vi "create.vi"(11 "tasks":refnum<class "task.lvclass">[](array[class])) -> (3 "sequence task out":refnum<class "sequence task.lvclass">)   [LabVIEW 2014, in "sequence task.lvclass"]
uses:
  sequence task.lvclass
  task/task.lvclass
  sequence task.lvclass/sequence task.ctl
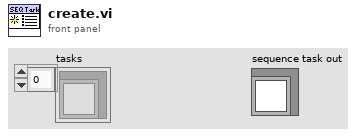
[diagram p1: front panel]
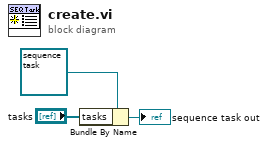
[diagram p0: block diagram]
diagram:
  n1 = Bundle By Name(cluster=refnum<class "sequence task.lvclass"> refnum ("function task in"), "tasks"="tasks") -> (→"sequence task out":refnum<class "sequence task.lvclass">)
